vi "ClusterEscala.vi"() -> ()   [LabVIEW 2020]
panel:
  out "Cluster 2":T1 {"Gauge" scale=0.0..50.0; "Slide" scale=0.0..100.0; "Thermometer" scale=0.0..100.0}
  in  "Cluster":T2
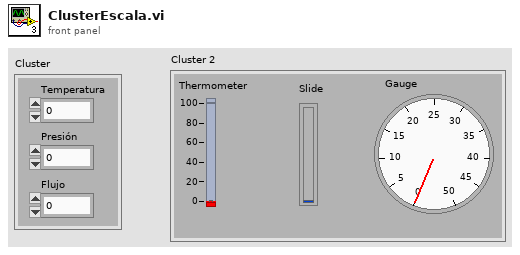
[diagram p1: front panel]
types:
  T1 = cluster{"Thermometer":dbl, "Slide":u8, "Gauge":dbl}
  T2 = cluster{"Temperatura":dbl, "Presión":dbl, "Flujo":dbl}
  T3 = cluster{"(°C/V)":i32, "(I/seg)/V":i32, "(N/m^2)/V":i32}
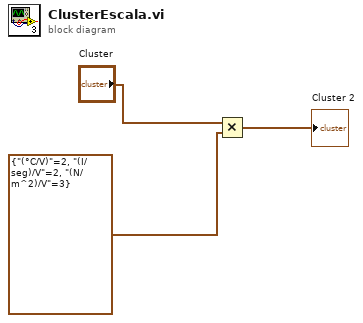
[diagram p0: block diagram]
diagram:
  n1 = Multiply(x="Cluster", y=T3 {"(°C/V)"=2, "(I/seg)/V"=2, "(N/m^2)/V"=3}) -> (x*y=→"Cluster 2":cluster{dbl, dbl, dbl})
